vi "MES操作函数H.vi"(3 "Tips":bool, 4 "TCP超时":u64=3000, 7 "SN":string="0105442MF011400002", 9 "MES字符串":string="0105442MF011400002", 10 "总结果（测试）":bool, 11 "MES配置":T1) -> (1 "状态":string)   [LabVIEW 2014]
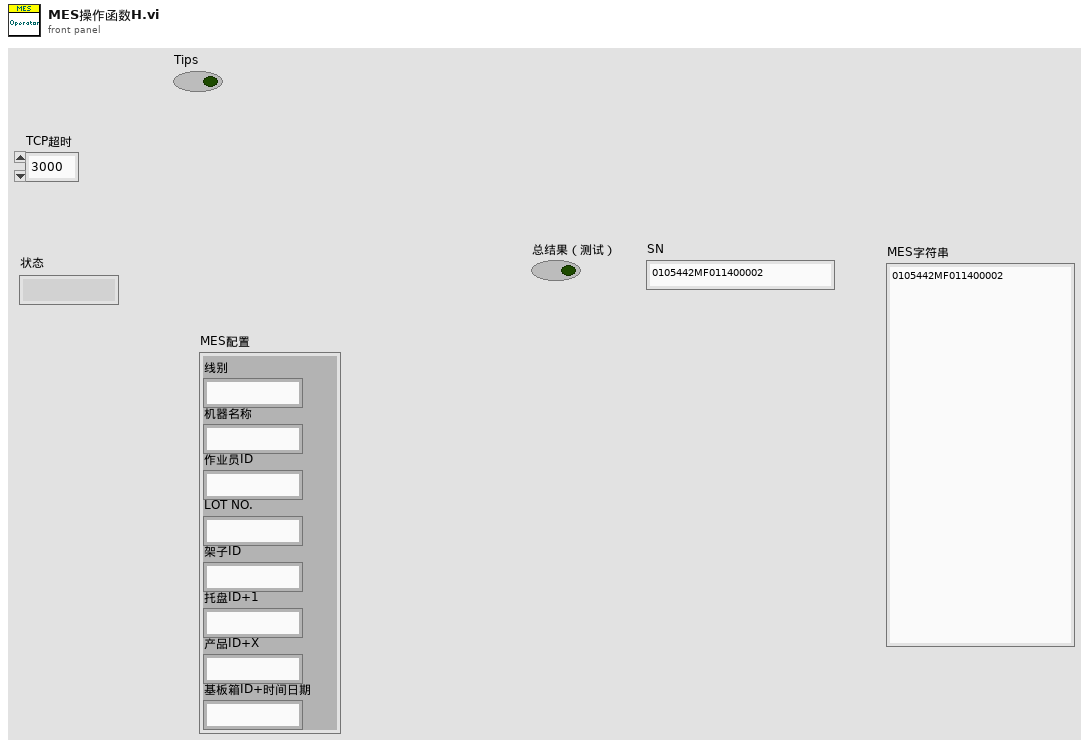
[diagram p1: front panel]
types:
  T1 = cluster{"线别":string, "机器名称":string, "作业员ID":string, "LOT NO.":string, "架子ID":string, "托盘ID+1":string, "产品ID+X":string, "基板箱ID+时间日期":string}
  T2 = enum16{"Left Button", "Center Button", "Right Button", "Window Close"}
  T3 = enum16{"open", "replace", "create", "open or create", "replace or create", "replace or create with confirmation"}
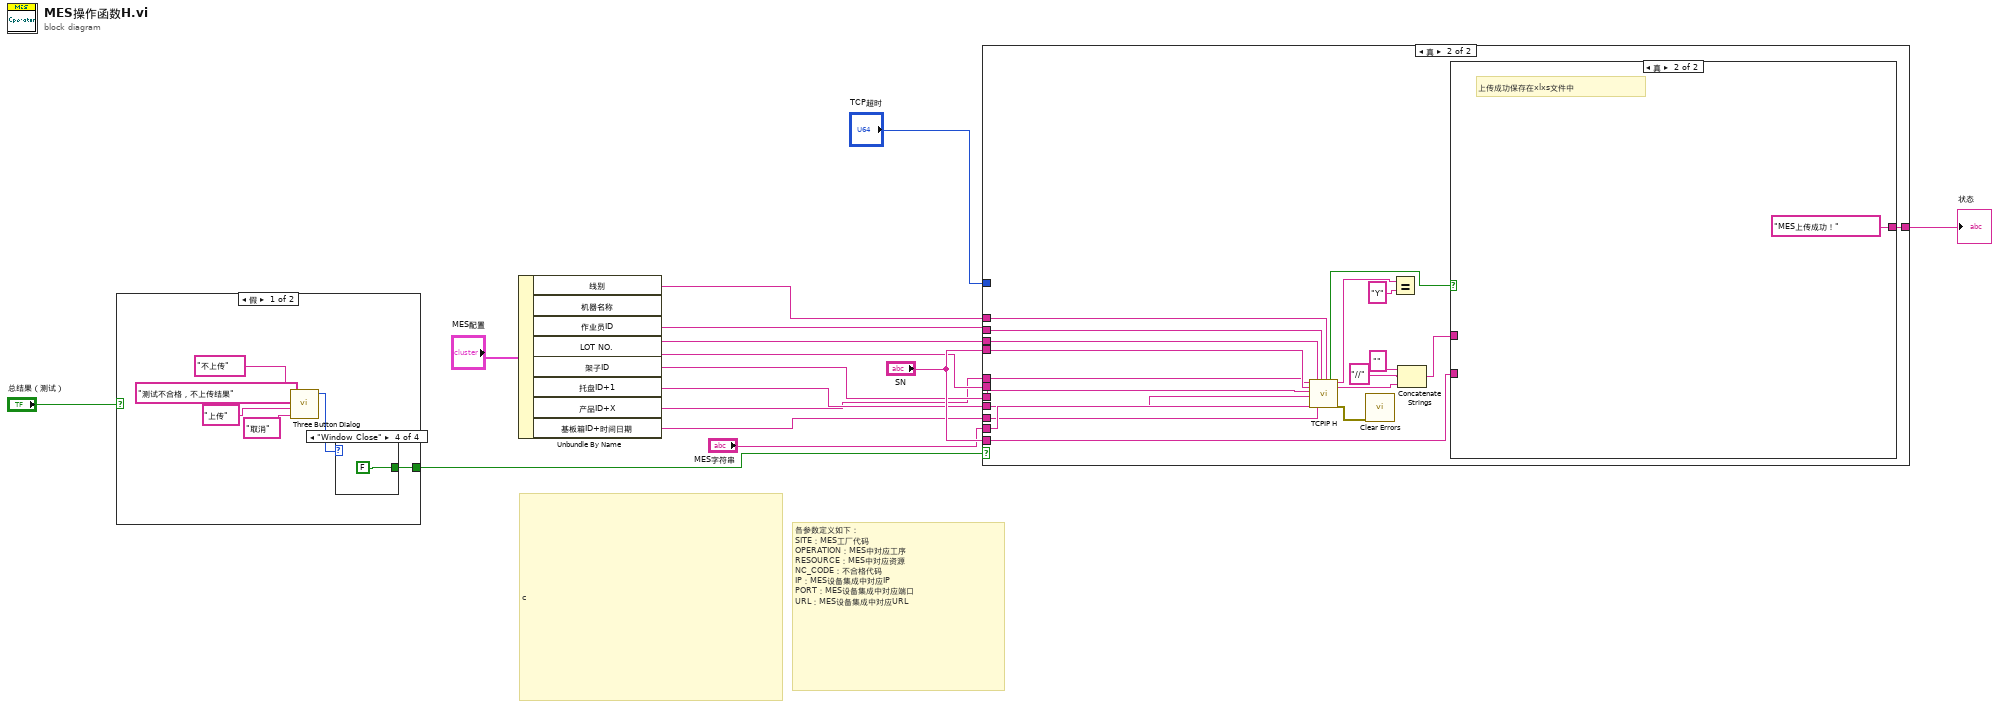
[diagram p0: block diagram]
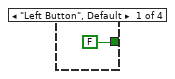
[diagram p2: hidden frame]
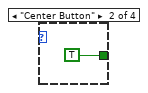
[diagram p3: hidden frame]
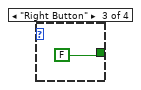
[diagram p4: hidden frame]
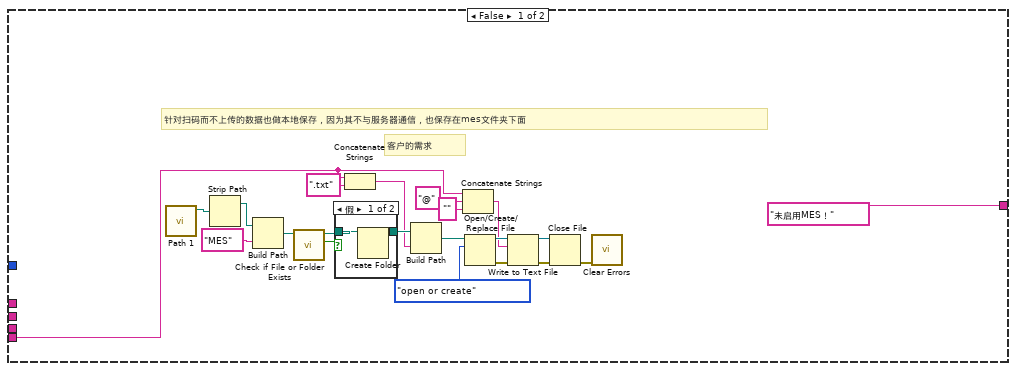
[diagram p6: hidden frame]
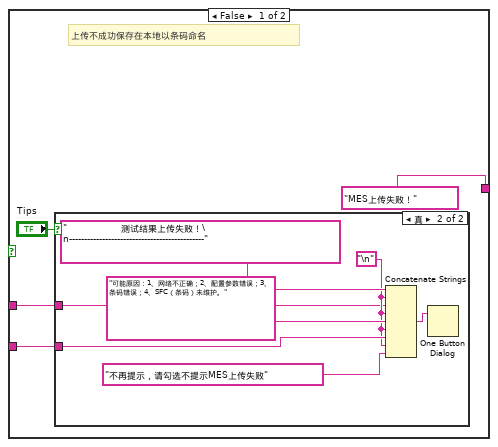
[diagram p8: hidden frame]
diagram:
  # "c"
  # "各参数定义如下：\nSITE：MES工厂代码\nOPERATION：MES中对应工序\nRESOURCE：MES中对应资源\nNC_CODE：不合格代码\nIP：MES设备集成中对应IP\nPORT：MES设备集成中对应端口\nURL：MES设备集成中对应URL"
  n1 = case shown="假" "总结果（测试）" {
    selector: "总结果（测试）" -> [_ w26]
    tunnel: [w16 w26] -> w2
    frame False {
      n2 = call <vilib>:"Three Button Dialog.vi"("Right Button Text (\"Cancel\")"="取消" ("Right Button Text (\"Cancel\")"), "Center Button Text (\"No\")"="上传" ("Center Button Text (\"No\")"), "Left Button Text (\"Yes\")"="不上传" ("Left Button Text (\"Yes\")"), "message"="测试不合格，不上传结果") -> ("Which Button?"=w17:T2)  [unwired: 7 in]
      n3 = case shown="\"Window Close\"" w17 {
        tunnel: [FALSE TRUE FALSE FALSE] -> w16
        frame "Left Button", Default {
        }
        frame "Center Button" {
        }
        frame "Right Button" {
        }
        frame "Window Close" {
        }
      }
    }
    frame True {
    }
  }
  n4 = Unbundle By Name("MES配置") -> ("线别"=w11:string, "机器名称"=w10:string, "作业员ID"=w5:string, "LOT NO."=w9:string, "架子ID"=w8:string, "托盘ID+1"=w7:string, "产品ID+X"=w1:string, "基板箱ID+时间日期"=w6:string)
  n5 = case shown="真" w2 {
    tunnel: "SN" -> [w29 w56]
    tunnel: "TCP超时" -> [_ _]
    tunnel: "SN" -> [_ w62]
    tunnel: ["未启用MES！" w61] -> w13
    tunnel: w11 -> [_ w59]
    tunnel: w10 -> [_ w58]
    tunnel: w9 -> [_ _]
    tunnel: w8 -> [_ w55]
    tunnel: w7 -> [_ w54]
    tunnel: w6 -> [_ w53]
    tunnel: w5 -> [_ w57]
    tunnel: "MES字符串" -> [_ w60]
    tunnel: w1 -> [_ w52]
    frame False {
      # "客户的需求"
      # "针对扫码而不上传的数据也做本地保存，因为其不与服务器通信，也保存在mes文件夹下面"
      n6 = call "Path 1.vi"() -> ("appended path"=w47:path)  [unwired: 11 in]
      n7 = Strip Path(path=w47) -> (stripped path=w46:path)  [unwired: 1 out]
      n8 = Build Path(base path=w46, name or relative path="MES" ("名称或相对路径")) -> (appended path=w44:path)
      n9 = call <vilib>:"Check if File or Folder Exists.vi"("path"=w44) -> ("file or folder exists?"=w43:bool, "dup path"=w42:path)  [unwired: 8 in, 1 out]
      n10 = case shown="假" w43 {
        tunnel: w42 -> [w48 w50]
        tunnel: [w49 w50] -> w41
        frame False {
          n11 = Create Folder(path (use dialog)=w48) -> (created path=w49:path)  [unwired: 2 in, 2 out]
        }
        frame True {
        }
      }
      n12 = Concatenate Strings(w29, ".txt" ("字符串")) -> (w31:string)
      n13 = Build Path(base path=w41, name or relative path=w31) -> (appended path=w40:path)
      n14 = Concatenate Strings(w29, "@" ("字符串"), "" ("字符串")) -> (w32:string)
      n15 = Open/Create/Replace File(file path (use dialog)=w40, operation (0:open)=T3."open or create" ("操作(0:open)")) -> (refnum out=w38:refnum<file>, error out=w37:errorcluster)  [unwired: 4 in, 1 out]
      n16 = Write to Text File(file (use dialog)=w38, text=w32, error in=w37) -> (refnum out=w35:refnum<file>, error out=w36:errorcluster)  [unwired: 1 in, 1 out]
      n17 = Close File(refnum=w35, error in=w36) -> (error out=w34:errorcluster)  [unwired: 1 out]
      n18 = call <vilib>:"Clear Errors.vi"("error in (no error)"=w34) -> ()  [unwired: 5 in, 2 out]
    }
    frame True {
      n19 = call "TCPIP H.vi"("产品ID+X 2"=w52, "LOT NO."=w56, "架子ID"=w55, "托盘ID+1"=w54, "MES字符串"=w60, "作业员ID"=w57, "基板箱ID+时间日期"=w53, "机器名称"=w58, "线别"=w59) -> ("x = y?"=w51:bool, "Y&N"=w64:string, "系统消息"=w69:string, "error out"=w66:errorcluster)  [unwired: 5 in, 2 out]
      n20 = call <vilib>:"Clear Errors.vi"("error in (no error)"=w66) -> ()  [unwired: 5 in, 2 out]
      n21 = Equal?(x=w64, y="Y") -> ()  [unwired: 1 out]
      n22 = Concatenate Strings("", "//" ("字符串"), w69) -> (w67:string)
      n23 = case shown="真" w51 {
        tunnel: w67 -> [w73 _]
        tunnel: w62 -> [w70 _]
        tunnel: ["MES上传失败！" ("字符串") "MES上传成功！" ("字符串")] -> w61
        frame False {
          # "上传不成功保存在本地以条码命名"
          n24 = case shown="真" "Tips" {
            tunnel: w73 -> [_ w74]
            tunnel: w70 -> [_ w77]
            frame False {
            }
            frame True {
              w76 = "\n"
              n25 = Concatenate Strings("                  测试结果上传失败！\n---------------------------------------------", w76, w74, w76, "可能原因：1、网络不正确；2、配置参数错误；3、条码错误；4、SFC（条码）未维护。" ("字符串"), w76, w77, w76, "不再提示，请勾选不提示MES上传失败" ("字符串")) -> (w80:string)
              n26 = One Button Dialog(message=w80) -> ()  [unwired: 1 in, 1 out]
            }
          }
        }
        frame True {
          # "上传成功保存在xlxs文件中"
        }
      }
    }
  }
  "状态" <- w13
